vi "Fields Get Measurements.vi"(8 "error in (no error)":errorcluster, 9 "Get Numerics only? (f)":bool, 10 "sDisplayName (empty, get all)":string, 11 "Connection Refnum":T1) -> (0 "error out":errorcluster, 2 "Measurement Fields":T2[](array[typedef]), 3 "dup Connection Refnum":T1, 4 "Data Present?":bool)   [LabVIEW 2011]
uses:
  Field Record.ctl
  Field DataTypes.ctl
  Field NextItem.ctl
  Summitek EXT/ODBC/SQL Controls/Connection Refnum.ctl
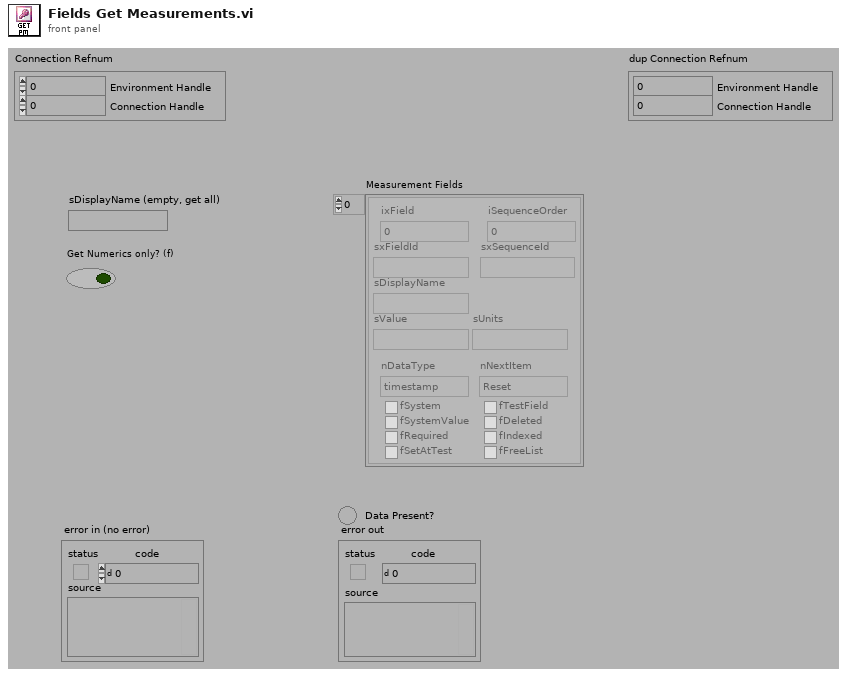
[diagram p1: front panel]
types:
  T1 = typedef "Connection Refnum.ctl" = cluster{"Environment Handle":i32, "Connection Handle":i32}
  T2 = typedef "Field Record.ctl" = cluster{"ixField":i32, "iSequenceOrder":i32, "sxFieldId":string, "sxSequenceId":string, "sDisplayName":string, "sValue":string, "sUnits":string, "nDataType":T3, "nNextItem":T4, "fSystem":bool, "fSystemValue":bool, "fRequired":bool, "fSetAtTest":bool, "fTestField":bool, "fDeleted":bool, "fIndexed":bool, "fFreeList":bool}
  T3 = typedef "Field DataTypes.ctl" = enum32{"text", "numeric", "list", "timestamp", "boolean"}
  T4 = typedef "Field NextItem.ctl" = enum32{"Reset", "Retain", "Auto-Increment"}
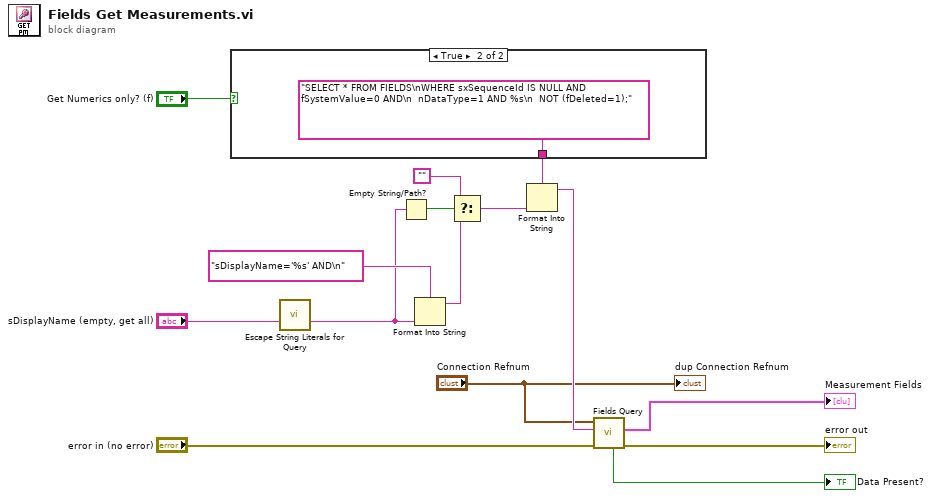
[diagram p0: block diagram]
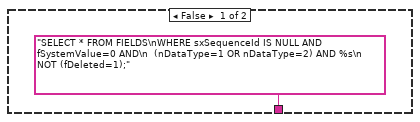
[diagram p2: hidden frame]
diagram:
  n1 = case shown="True" "Get Numerics only? (f)" {
    tunnel: ["SELECT * FROM FIELDS\nWHERE sxSequenceId IS NULL AND fSystemValue=0 AND\n  (nDataType=1 OR nDataType=2) AND %s\n  NOT (fDeleted=1);" ("Query Name") "SELECT * FROM FIELDS\nWHERE sxSequenceId IS NULL AND fSystemValue=0 AND\n  nDataType=1 AND %s\n  NOT (fDeleted=1);" ("Query Name")] -> w12
    frame False {
    }
    frame True {
    }
  }
  n2 = call "Escape String Literals for Query.vi"("String"="sDisplayName (empty, get all)") -> ("escaped String"=w8:string)  [unwired: 1 in, 13 out]
  n3 = Empty String/Path?(string/path=w8) -> (empty?=w9:bool)
  n4 = Format Into String(format string="sDisplayName='%s' AND\n" ("Query Name"), w8) -> (resulting string=w7:string)  [unwired: 2 in, 1 out]
  n5 = Select(t="", s=w9, f=w7) -> (s? t:f=w6:string)
  n6 = Format Into String(format string=w12, w6) -> (resulting string=w11:string)  [unwired: 2 in, 1 out]
  n7 = call "Fields Query.vi"("error in (no error)"="error in (no error)", "Query"=w11, "Connection Refnum"="Connection Refnum") -> ("error out"=→"error out":errorcluster, "Fields"=→"Measurement Fields":T2[], "Data Present?"=→"Data Present?":bool)  [unwired: 2 in, 4 out]
  "dup Connection Refnum" <- "Connection Refnum"
